vi "Concatenate Strings.vi"() -> ()   [LabVIEW 2020]
doc: "This example shows how the Concatenate Strings function operates with different types of data."
panel:
  in  "Tab Control":T1(tab)
  out "Concatenated String":string
  in  "String 3":string="Concatenated"
  in  "String 2":string="Be"
  in  "String 1":string="To"
  out "Concatenated Array":string
  in  "Array":string[](array[string])=["Array", "Of", "Strings"]
  out "Concatenated String":string
  in  "String":string="d"
  in  "Array":string[](array[string])=["Array", "Of", "Strings"]
  # "Overview: Demonstrates how the Concatenate Strings function operates with different data types.\nInstructions:\n1. Run the VI.\n2. Examine the different cases."
  # "The most common use of the Concatenate Strings function is to combine several individual strings into one string."
  # "When an array of strings is wired to the Concatenate Strings functions, all the strings in the array are combined into one string."
  # "When both arrays and scalar strings are wired to the Concatenate Strings function, all the strings in the arrays, and the scalar strings, are combined into one string."
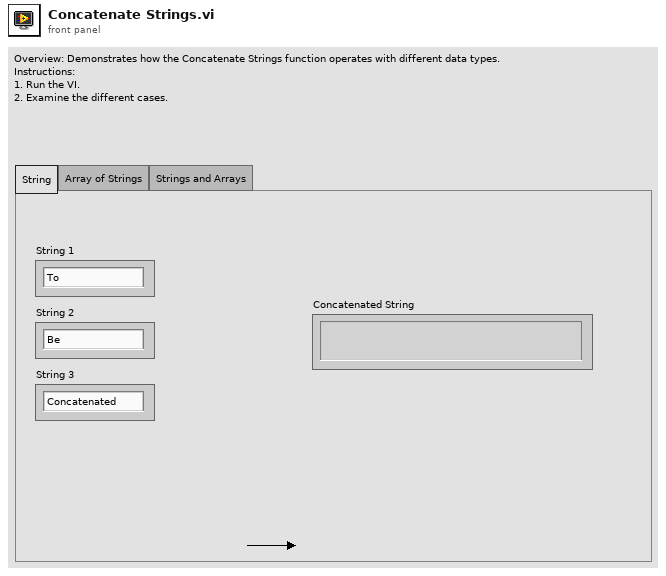
[diagram p1: front panel]
types:
  T1 = enum32{"String", "Array of Strings", "Strings and Arrays"}
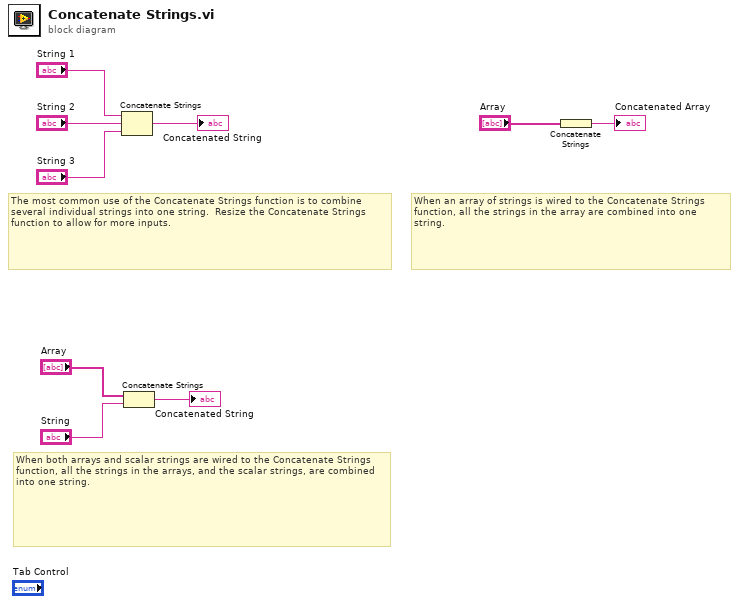
[diagram p0: block diagram]
diagram:
  # "The most common use of the Concatenate Strings function is to combine several individual strings into one string.  Resize the Concatenate Strings function to allow for more inputs."
  # "When an array of strings is wired to the Concatenate Strings function, all the strings in the array are combined into one string."
  # "When both arrays and scalar strings are wired to the Concatenate Strings function, all the strings in the arrays, and the scalar strings, are combined into one string."
  n1 = Concatenate Strings("String 1", "String 2", "String 3") -> (→"Concatenated String":string)
  n2 = Concatenate Strings("Array", "String") -> (→"Concatenated String":string)
  n3 = Concatenate Strings("Array") -> (→"Concatenated Array":string)
